vi "Loop.vi"(11 "TEMPLATE Queue in":refnum<class "TEMPLATE Queue.lvclass">) -> (3 "TEMPLATE Queue out":refnum<class "TEMPLATE Queue.lvclass">)   [LabVIEW 2021, in "_Template.lvlib" / "Templates.lvlib" / "TEMPLATE Queue.lvlib" / "TEMPLATE Queue.lvclass"]
uses:
  TEMPLATE Queue.lvclass
  C:/Program Files/National Instruments/LabVIEW 2021/vi.lib/Nathan Davis/jettl/jettl/jettl/jettl.lvclass
  <vilib>/Nathan Davis/jettl/jettl/Msg Strategy/Msg Strategy.lvclass
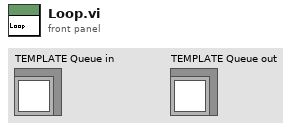
[diagram p1: front panel]
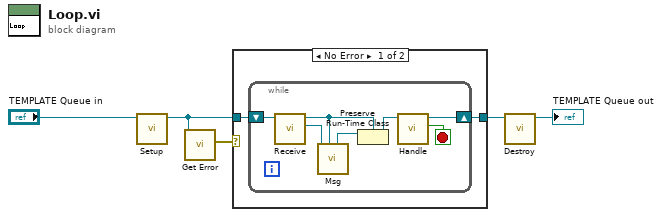
[diagram p0: block diagram]
diagram:
  n1 = call-dynamic "Setup.vi"("TEMPLATE Queue in"="TEMPLATE Queue in") -> ("TEMPLATE Queue out"=w1:refnum<class "TEMPLATE Queue.lvclass">)  [unwired: 10 in]
  n2 = call-dynamic "Get Error.vi"("TEMPLATE Queue in"=w1) -> ("Error"=w3:errorcluster)  [unwired: 10 in]
  n3 = case shown="No Error" w3 {
    tunnel: [w7 w15] -> w2
    tunnel: w1 -> [w6 w15]
    frame No Error {
      n4 = while {
        shift-right: [w10] -> w7
        shift-left: w6 -> [w14]
        stop <- w9 stop-if-true
        n5 = call-dynamic "Receive.vi"("TEMPLATE Queue in"=w14) -> ("Msg Strategy"=w12:refnum<class "Msg Strategy.lvclass">, "TEMPLATE Queue out"=w11:refnum<class "TEMPLATE Queue.lvclass">)  [unwired: 9 in]
        n6 = call-dynamic "Msg.vi"("jettl in"=w11, "Msg Strategy in"=w12) -> ("jettl out"=w13:refnum<class "jettl.lvclass">)  [unwired: 9 in]
        n7 = Preserve Run-Time Class(object in=w13, 2:w11) -> (object out=w8:refnum<class "TEMPLATE Queue.lvclass">)  [unwired: 1 in, 1 out]
        n8 = call-dynamic "Handle.vi"("TEMPLATE Queue in"=w8) -> ("Destroy?"=w9:bool, "TEMPLATE Queue out"=w10:refnum<class "TEMPLATE Queue.lvclass">)  [unwired: 9 in]
      }
    }
    frame Error {
    }
  }
  n9 = call-dynamic "Destroy.vi"("TEMPLATE Queue in"=w2) -> ("TEMPLATE Queue out"=→"TEMPLATE Queue out":refnum<class "TEMPLATE Queue.lvclass">)  [unwired: 10 in]
